vi "Mod_OFDM_Config_OFDM_Symbol_Range_Properties.vi"(1 "OFDM PARAMETERS":T2={"# of Sub Carrier"=64, "Length Of Cylic Prefix"=16}, 11 "error in":errorcluster) -> (13 "Data Range":T1, 15 "error out":errorcluster)   [LabVIEW 2010]
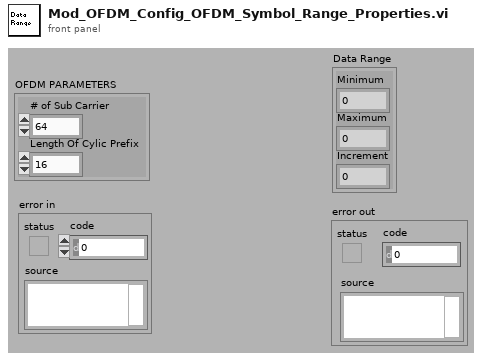
[diagram p1: front panel]
types:
  T1 = cluster{"Minimum":i32, "Maximum":i32, "Increment":i32}
  T2 = cluster{"# of Sub Carrier":i32, "Length Of Cylic Prefix":i32}
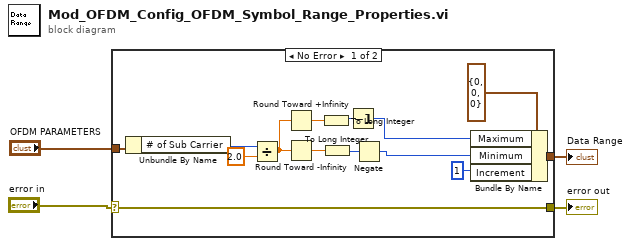
[diagram p0: block diagram]
diagram:
  n1 = case shown="No Error" "error in" {
    selector: "error in" -> [w5 w19]
    tunnel: "OFDM PARAMETERS" -> [w18 _]
    tunnel: [w6 _] -> w3
    tunnel: [w5 w19] -> w1
    frame No Error {
      n2 = Unbundle By Name(w18) -> ("# of Sub Carrier"=w17:i32)
      n3 = Divide(x=w17, y=2.0) -> (x/y=w15:dbl)
      n4 = Round Toward +Infinity(x=w15) -> (ceil(x): smallest int >= x=w14:dbl)
      n5 = Round Toward -Infinity(1:w15) -> (0:w13:dbl)
      n6 = To Long Integer(number=w14) -> (32bit integer=w12:i32)
      n7 = To Long Integer(number=w13) -> (32bit integer=w11:i32)
      n8 = Decrement(x=w12) -> (x-1=w9:i32)
      n9 = Negate(x=w11) -> (-x=w8:i32)
      n10 = Bundle By Name(cluster=T1 {"Minimum"=0, "Maximum"=0, "Increment"=0} ("Data Range"), "Maximum"=w9, "Minimum"=w8, "Increment"=1) -> (w6:T1)
    }
    frame Error {
    }
  }
  "error out" <- w1
  "Data Range" <- w3
